vi "Test Ordered Hash.vi"   [LabVIEW 2012]
uses:
  <vilib>/Utility/config.llb/NI_LVConfig.lvlib
types:
  T1 = typedef "NI_LVConfig.lvlib/Config Data RefNum.ctl" = refnum<k1>
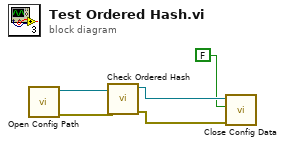
[diagram p0: block diagram]
diagram:
  n1 = call "Open Config Path.vi"() -> ("error out"=w4:errorcluster, "cfg_ref out"=w5:T1)  [unwired: 10 in]
  n2 = call "Check Ordered Hash.vi"("error in"=w4, "refnum"=w5) -> ("error out"=w2:errorcluster, "refnum out"=w3:T1)  [unwired: 7 in, 1 out]
  n3 = call <vilib>:"Close Config Data.vi"("error in (no error)"=w2, "write file if changed (T)"=FALSE, "refnum"=w3) -> ()  [unwired: 7 in, 2 out]
